vi "Convert U32 to byte array.vi"(1 "U32 in":i32) -> (0 "Array of 4 bytes out":u8[](array[numeric]))   [LabVIEW 2018, in "LV-Julia_ZMQ-Roundtrip_lib.lvlib"]
uses:
  LV-Julia_ZMQ-Roundtrip_lib.lvlib
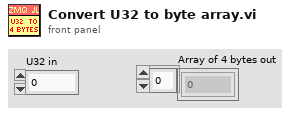
[diagram p1: front panel]
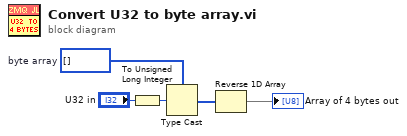
[diagram p0: block diagram]
diagram:
  w3 = u8[] []  # byte array
  n1 = To Unsigned Long Integer(number="U32 in") -> (unsigned 32bit integer=w2:u32)
  n2 = Type Cast(type=w3, x=w2) -> (*(type *) &x=w4:u8[])
  n3 = Reverse 1D Array(array=w4) -> (reversed array=→"Array of 4 bytes out":u8[])
